vi "Read Module Reference.vi"(8 "error in":errorcluster, 11 "Shared Resources in":refnum<class "Shared Resources.lvclass">) -> (0 "error out":errorcluster, 2 "module reference":T1, 3 "Shared Resources out":refnum<class "Shared Resources.lvclass">)   [LabVIEW 2020, in "AIM MIL-STD-1553 Engine.lvlib" / "Implementation.lvlib" / "Shared Resources.lvclass"]
uses:
  Shared Resources.lvclass
  Shared Resources.lvclass/Shared Resources.ctl
  Hardware API/Init Board/Module Reference.ctl
  Hardware API/AIM MIL-STD-1553 Hardware API.lvlib
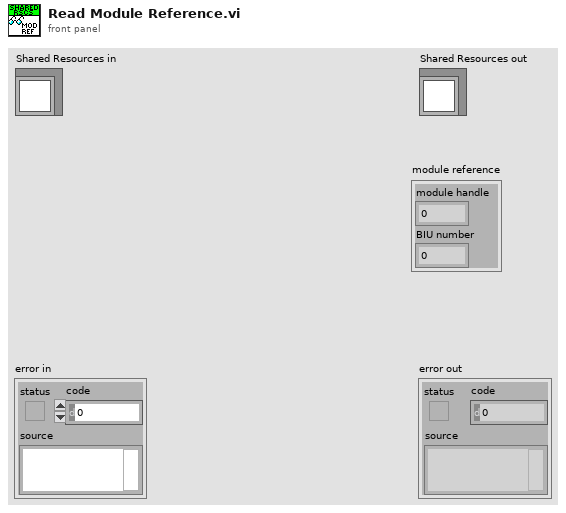
[diagram p1: front panel]
types:
  T1 = typedef "AIM MIL-STD-1553 Hardware API.lvlib/Module Reference.ctl" = cluster{"module handle":u32, "BIU number":u8}
  T2 = typedef "AIM MIL-STD-1553 Wrapped Palette.lvlib/Module Reference.ctl" = cluster{"module handle":u32, "BIU number":u8}
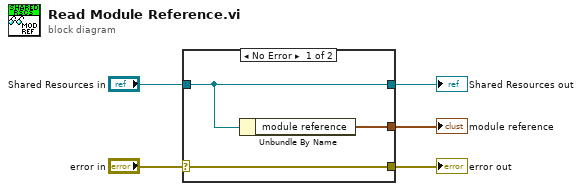
[diagram p0: block diagram]
diagram:
  n1 = case shown="No Error" "error in" {
    selector: "error in" -> [w8 w9]
    tunnel: [w8 w9] -> w4
    tunnel: [w7 w10] -> w2
    tunnel: "Shared Resources in" -> [w7 w10]
    tunnel: [w6 _] -> w1
    frame No Error {
      n2 = Unbundle By Name(w7) -> ("module reference"=w6:T2)
    }
    frame Error {
    }
  }
  "error out" <- w4
  "Shared Resources out" <- w2
  "module reference" <- w1
